vi "DATA SAVE.vi"(5 "save":bool=TRUE, 7 "tdms ref":refnum<k34>, 8 "error in":errorcluster, 10 "Wave":waveform(dbl)[](array[waveform])) -> (0 "error out":errorcluster caption="错误输出")   [LabVIEW 2016]
panel:
  out "Time Used":u32
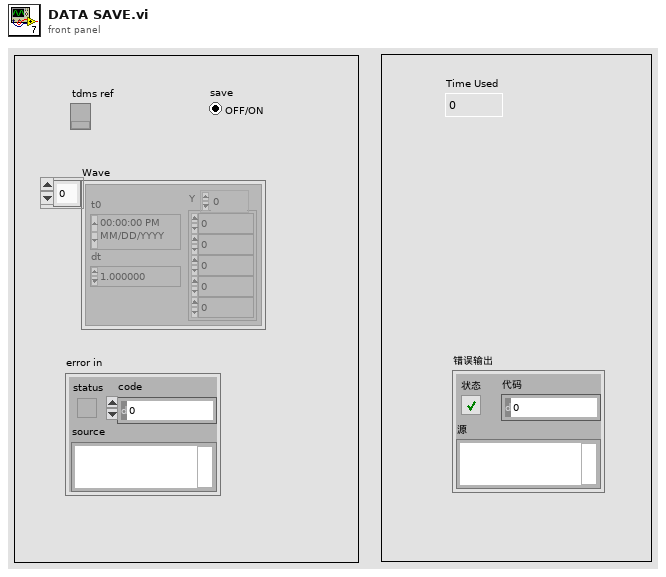
[diagram p1: front panel]
types:
  T1 = cluster{"Queue Name":string, "DAQ Channels":string[], "Queue Type":string}[]
  T2 = cluster{"Queue Name":string, "DAQ Channels":string[], "Queue Type":string}
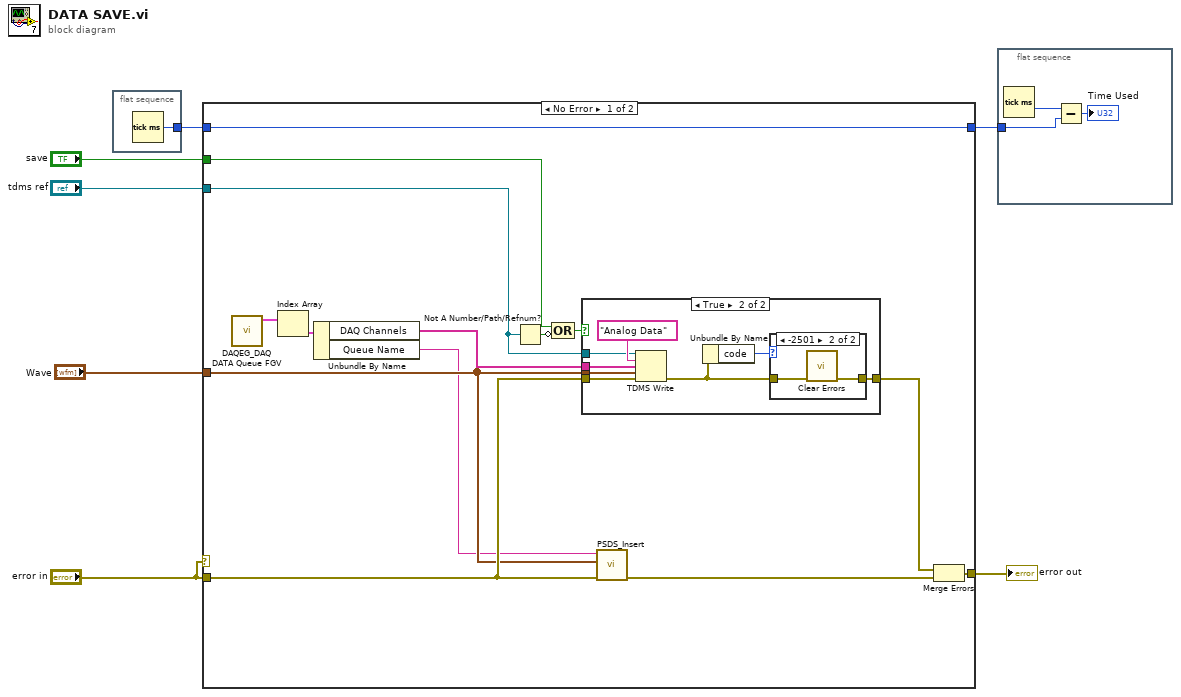
[diagram p0: block diagram]
diagram:
  n1 = flat-sequence {
    tunnel: [w8] -> w4
    frame #0 {
      n2 = Tick Count (ms)() -> (millisecond timer value=w8:u32)
    }
  }
  n3 = case shown="No Error" "error in" {
    tunnel: [w20 w36] -> w7
    tunnel: "save" -> [w19 _]
    tunnel: "tdms ref" -> [w17 _]
    tunnel: "error in" -> [w14 w36]
    tunnel: w4 -> [w15 w35]
    tunnel: [w15 w35] -> w3
    tunnel: "Wave" -> [w13 _]
    frame No Error {
      n4 = call "DAQEG_DAQ DATA Queue FGV.vi"() -> ("DAQ DATA Out"=w12:T1)  [unwired: 10 in, 1 out]
      n5 = Index Array(array=w12) -> (element=w11:T2)  [unwired: 1 in]
      n6 = Unbundle By Name(w11) -> ("DAQ Channels"=w10:string[], "Queue Name"=w9:string)
      n7 = Not A Number/Path/Refnum?(number/path/refnum=w17) -> (NaN/Path/Refnum?=w16:bool)
      n8 = Compound Arithmetic op=OR(w19, invert w16) -> (w18:bool)
      n9 = case shown="True" w18 {
        tunnel: w13 -> [_ w31]
        tunnel: w10 -> [_ w29]
        tunnel: w14 -> [w23 w28]
        tunnel: [w23 w24] -> w21
        tunnel: w17 -> [_ w27]
        frame False {
        }
        frame True {
          n10 = TDMS Write(0:w27, 5:"Analog Data" ("组名称输入（无标题）"), 7:w29, 9:w31, 11:w28) -> (15:w26:errorcluster)  [unwired: 1 in, 3 out]
          n11 = Unbundle By Name(w26) -> ("code"=w25:i32)
          n12 = case shown="-2501" w25 {
            tunnel: w26 -> [w32 w34]
            tunnel: [w32 w33] -> w24
            frame 0, Default {
            }
            frame -2501 {
              n13 = call <vilib>:"Clear Errors.vi"("error in (no error)"=w34) -> ("error out"=w33:errorcluster)  [unwired: 5 in, 1 out]
            }
          }
        }
      }
      n14 = call "PSDS_Insert.vi"("error in (no error)"=w14, "Wave"=w13, "Object Name"=w9) -> ("error out"=w22:errorcluster)  [unwired: 7 in, 1 out]
      n15 = Merge Errors(w21, w22) -> (w20:errorcluster)
    }
    frame Error {
    }
  }
  "error out" <- w7
  n16 = flat-sequence {
    tunnel: w3 -> [w38]
    frame #0 {
      n17 = Tick Count (ms)() -> (millisecond timer value=w39:u32)
      n18 = Subtract(x=w39, y=w38) -> (x-y=→"Time Used":u32)
    }
  }
